vi "Msg and Actor Read.vi"(9 "Tree":string(tree), 10 "Tree Ref":refnum<vi>) -> (1 "Name":string, 2 "Type":T1)   [LabVIEW 2025, in "_Shared.lvlib" / "Tree.lvlib"]
uses:
  Tree.lvlib
  Type.ctl
  _Shared.lvlib
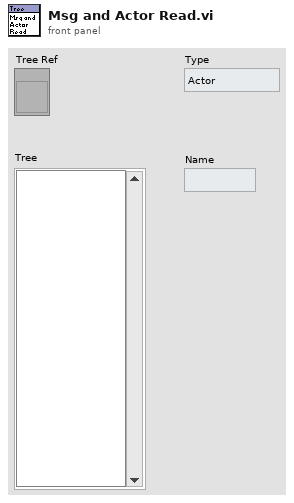
[diagram p1: front panel]
types:
  T1 = typedef "_Shared.lvlib/Type.ctl" = enum16{"Actor", "Msg"}
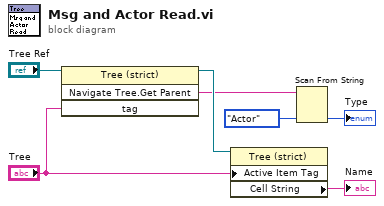
[diagram p0: block diagram]
diagram:
  n1 = invoke class="Tree (strict)" method="Navigate Tree.Get Parent"(reference="Tree Ref", "tag"="Tree") -> (reference out=w4:refnum<vi>, "Navigate Tree:Get Parent"=w2:string)  [unwired: 2 in, 2 out]
  n2 = property class="Tree (strict)"(reference=w4, "Active Item Tag"="Tree") -> ("Cell String"=→"Name":string)  [unwired: 1 in, 2 out]
  n3 = Scan From String(input string=w2, default 1=Type."Actor" ("Type")) -> (output 1=→"Type":T1)  [unwired: 3 in, 3 out]
